vi "Initialization VI.vi"(8 "error in (no error)":errorcluster, 10 "Custom XML":string, 11 "Device Item Ref in":T1 format="%.0x") -> (0 "error out":errorcluster, 3 "Device Item Ref out":T1 format="%.0x")   [LabVIEW 2021, in "Modbus Master System Explorer.lvlib"]
uses:
  Modbus Master System Explorer.lvlib
  <vilib>/NI VeriStand/Custom Device API/Custom Device Item Ref.ctl
  Shared/Controls/Interface Type.ctl
  Shared/Controls/Serial Type.ctl
  Shared/Controls/Flow Control.ctl
  Shared/Controls/Parity.ctl
  SubVIs/Radix.ctl
  Shared/Write Mode.ctl
  Shared/Constants.vi
  <vilib>/NI VeriStand/Custom Device API/Set Item Property (U16).vi
  <vilib>/NI VeriStand/Custom Device API/Set Item Property (I32).vi
  <vilib>/NI VeriStand/Custom Device API/Custom Device API.lvlib
  Shared/Modbus Master Shared.lvlib
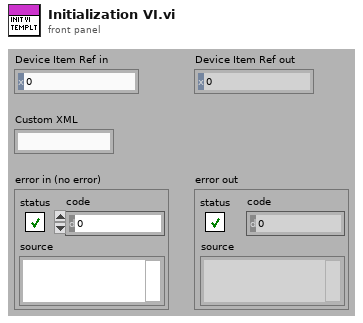
[diagram p1: front panel]
types:
  T1 = typedef "Custom Device API.lvlib/Custom Device Item Ref.ctl" = u64
  T2 = typedef "Modbus Master Shared.lvlib/Write Mode.ctl" = enum16{"Value Change", "Interval"}
  T3 = typedef "Modbus Master System Explorer.lvlib/Radix.ctl" = enum32{"Decimal", "Hexidecimal"}
  T4 = typedef "Modbus Master Shared.lvlib/Serial Type.ctl" = enum16{"RTU", "ASCII"}
  T5 = typedef "Modbus Master Shared.lvlib/Interface Type.ctl" = enum16{"TCP Master", "Serial Master", "TCP Slave", "Serial Slave"}
  T6 = typedef "Modbus Master Shared.lvlib/Parity.ctl" = u16
  T7 = typedef "Modbus Master Shared.lvlib/Flow Control.ctl" = u16
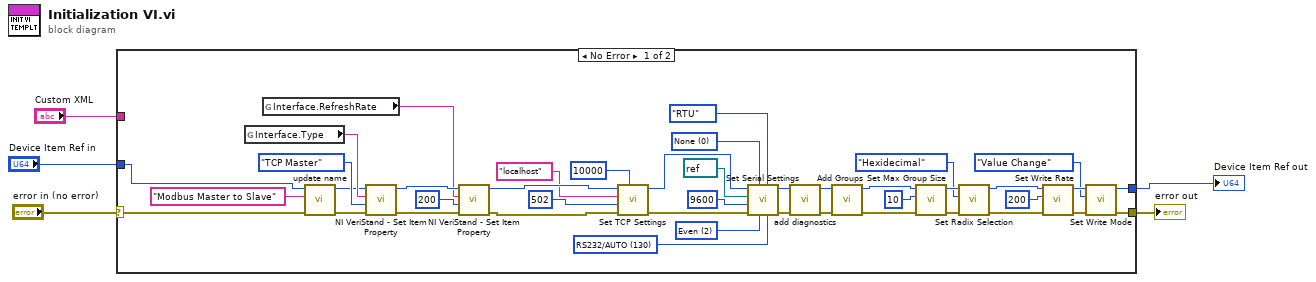
[diagram p0: block diagram]
diagram:
  n1 = case shown="No Error" "error in (no error)" {
    selector: "error in (no error)" -> [w31 w49]
    tunnel: [w9 w49] -> w5
    tunnel: [w8 w48] -> w3
    tunnel: "Device Item Ref in" -> [w32 w48]
    tunnel: "Custom XML" -> [_ _]
    frame No Error {
      w14 = i16 130 items=["Unknown"=-1, "RS485/Wire4"=0, "RS485/Wire2-EchoDTR"=1, "RS485/Wire2-CtrlDTR"=2, "RS485/Wire2-Auto"=3, "RS232/DTE"=128, "RS232/DCE"=129, "RS232/AUTO"=130] ("Wire Mode")
      w36 = T6 2 items=["None", "Odd", "Even", "Mark", "Space"] ("parity (even)")
      w40 = T7 0 items=["None", "XON/XOFF", "RTS/CTS", "XON/XOFF & RTS/CTS", "DTR/DSR", "XON/XOFF & DTR/DSR"] ("flow control (none)")
      n2 = global read "Constants.vi" "Interface.Type"() -> (w47:string)
      n3 = global read "Constants.vi" "Interface.RefreshRate"() -> (w27:string)
      n4 = call "update name.vi"("error in (no error)"=w31, "Desired Alias"="Modbus Master to Slave", "Parent Ref in"=w32) -> ("error out"=w37:errorcluster, "Parent Ref dup"=w34:T1)  [unwired: 7 in]
      n5 = call-poly <vilib>:"NI VeriStand - Set Item Property.vi"("error in (no error)"=w37, "Value"=Interface_Type."TCP Master" ("Interface Type"), "Property Name"=w47, "Item Ref in"=w34) -> ("error out"=w29:errorcluster, "Item Ref out"=w30:T1)  [unwired: 5 in, 1 out]
      n6 = call-poly <vilib>:"NI VeriStand - Set Item Property.vi"("error in (no error)"=w29, "Value"=200, "Property Name"=w27, "Item Ref in"=w30) -> ("error out"=w28:errorcluster, "Item Ref out"=w46:T1)  [unwired: 5 in, 1 out]
      n7 = call "Set TCP Settings.vi"("Timeout"=10000, "error in (no error)"=w28, "Port"=u16 502 ("Value"), "Address"="localhost" ("Value"), "Item Ref in"=w46) -> ("error out"=w43:errorcluster, "Item Ref out"=w42:T1)  [unwired: 5 in]
      n8 = call "Set Serial Settings.vi"("Wire Mode"=w14, "serial type"=Serial_Type."RTU", "parity (even)"=w36, "flow control (none)"=w40, "error in (no error)"=w43, "baud rate"=u32 9600, "VISA resource name"=refnum<visa-resource-name> refnum, "Item Ref in"=w42) -> ("error out"=w24:errorcluster, "Item Ref out"=w25:T1)  [unwired: 2 in]
      n9 = call "add diagnostics.vi"("error in (no error)"=w24, "Item Ref in"=w25) -> ("error out"=w22:errorcluster, "Parent Ref out"=w23:T1)  [unwired: 8 in]
      n10 = call "Add Groups.vi"("error in (no error)"=w22, "Item Ref in"=w23) -> ("error out"=w19:errorcluster, "Item Ref out"=w20:T1)  [unwired: 8 in]
      n11 = call "Set Max Group Size.vi"("error in (no error)"=w19, "Value"=10, "Item Ref in"=w20) -> ("error out"=w16:errorcluster, "Item Ref out"=w17:T1)  [unwired: 7 in]
      n12 = call "Set Radix Selection.vi"("error in (no error)"=w16, "Radix"=Radix."Hexidecimal", "Item Ref in"=w17) -> ("error out"=w10:errorcluster, "Item Ref out"=w11:T1)  [unwired: 7 in]
      n13 = call "Set Write Rate.vi"("error in (no error)"=w10, "Value"=200, "Item Ref in"=w11) -> ("error out"=w12:errorcluster, "Item Ref out"=w13:T1)  [unwired: 7 in]
      n14 = call "Set Write Mode.vi"("error in (no error)"=w12, "Write Mode"=Write_Mode."Value Change", "Item Ref in"=w13) -> ("error out"=w9:errorcluster, "Item Ref out"=w8:T1)  [unwired: 7 in]
    }
    frame Error {
    }
  }
  "error out" <- w5
  "Device Item Ref out" <- w3
